vi "Individual Tube ON - OFF.vi"(6 "Single Tube ON/OFF":bool, 7 "Tube #":i32 min=0 max=63) -> ()   [LabVIEW 2020]
uses:
  <vilib>/DAQmx/write.llb/DAQmx Write (Digital U8 1Chan 1Samp).vi
  <vilib>/DAQmx/create/channels.llb/DAQmx Create Channel (DO-Digital Output).vi
  <vilib>/DAQmx/miscellaneous.llb/DAQmx Fill In Error Info.vi
panel:
  out "Status(U8) 2":u8
  in  "lines 2":tag="Dev2/port0/line0:7"
  out "Status(U8)":u8
  in  "lines":tag="Dev2/port0/line0:7"
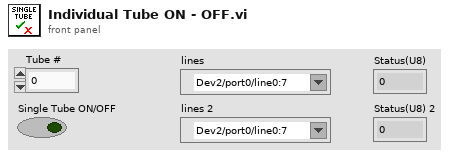
[diagram p1: front panel]
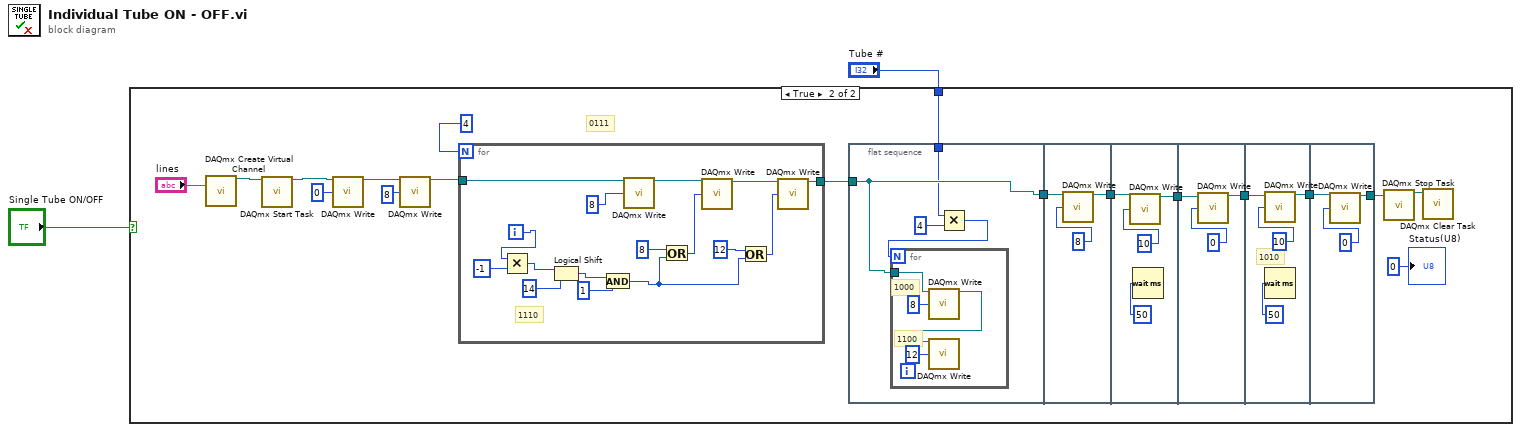
[diagram p0: block diagram]
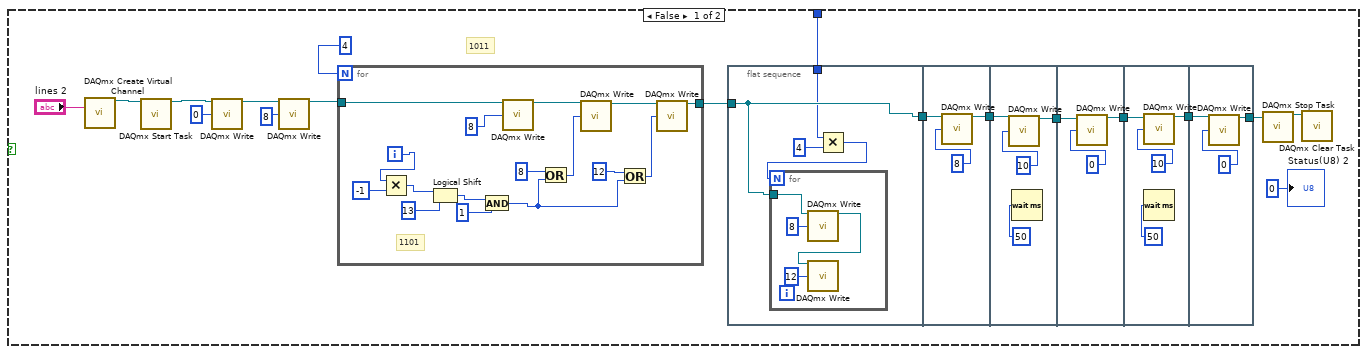
[diagram p2: hidden frame]
diagram:
  n1 = case shown="True" "Single Tube ON/OFF" {
    tunnel: "Tube #" -> [w3 w62]
    frame False {
      # "1011"
      n2 = call-poly <vilib>:"DAQmx Create Virtual Channel.vi"("lines"="lines 2") -> ("task out"=w15:refnum<k21>)  [unwired: 13 in, 1 out]
      n3 = call <vilib>:"DAQmx Start Task.vi"("task/channels in"=w15) -> ("task out"=w9:refnum<k21>)  [unwired: 13 in, 1 out]
      n4 = call-poly <vilib>:"DAQmx Write.vi"("task/channels in"=w9, "data"=u8 0) -> ("task out"=w8:refnum<k21>)  [unwired: 11 in, 2 out]
      n5 = call-poly <vilib>:"DAQmx Write.vi"("task/channels in"=w8, "data"=u8 8) -> ("task out"=w11:refnum<k21>)  [unwired: 11 in, 2 out]
      n6 = for {
        N: 4 -> [_]
        tunnel: w11 -> [w50]
        tunnel: [w47] -> w5
        i -> [w59]
        # "1101"
        n7 = Multiply(x=w59, y=-1) -> (x*y=w57:i32)
        n8 = Logical Shift(y=w57, x=u8 13) -> (x << y=w61:u8)
        n9 = And(x=w61, y=u32 1) -> (x .and. y?=w53:u32)
        n10 = call-poly <vilib>:"DAQmx Write.vi"("task/channels in"=w50, "data"=u32 8 ("x")) -> ("task out"=w49:refnum<k21>)  [unwired: 11 in, 2 out]
        n11 = Or(x=u32 8, y=w53) -> (x .or. y?=w54:u32)
        n12 = call-poly <vilib>:"DAQmx Write.vi"("task/channels in"=w49, "data"=w54) -> ("task out"=w48:refnum<k21>)  [unwired: 11 in, 2 out]
        n13 = Or(x=u32 12, y=w53) -> (x .or. y?=w51:u32)
        n14 = call-poly <vilib>:"DAQmx Write.vi"("task/channels in"=w48, "data"=w51) -> ("task out"=w47:refnum<k21>)  [unwired: 11 in, 2 out]
      }
      n15 = flat-sequence {
        tunnel: [w22] -> w20
        tunnel: w5 -> [w22]
        tunnel: w3 -> [w21]
        tunnel: [w29] -> w19
        tunnel: w20 -> [w30]
        tunnel: w19 -> [w33]
        tunnel: [w32] -> w18
        tunnel: w18 -> [w37]
        tunnel: [w36] -> w17
        tunnel: w17 -> [w40]
        tunnel: [w39] -> w16
        tunnel: w16 -> [w44]
        tunnel: [w43] -> w6
        frame #0 {
          n16 = Multiply(x=w21, y=4) -> (x*y=w24:i32)
          n17 = for {
            N: w24 -> [_]
            tunnel: w22 -> [w26]
            n18 = call-poly <vilib>:"DAQmx Write.vi"("task/channels in"=w26, "data"=u8 8) -> ("task out"=w25:refnum<k21>)  [unwired: 11 in, 2 out]
            n19 = call-poly <vilib>:"DAQmx Write.vi"("task/channels in"=w25, "data"=u8 12) -> ()  [unwired: 11 in, 3 out]
          }
        }
        frame #1 {
          n20 = call-poly <vilib>:"DAQmx Write.vi"("task/channels in"=w30, "data"=u8 8) -> ("task out"=w29:refnum<k21>)  [unwired: 11 in, 2 out]
        }
        frame #2 {
          n21 = call-poly <vilib>:"DAQmx Write.vi"("task/channels in"=w33, "data"=u8 10) -> ("task out"=w32:refnum<k21>)  [unwired: 11 in, 2 out]
          n22 = Wait (ms)(milliseconds to wait=u32 50) -> ()  [unwired: 1 out]
        }
        frame #3 {
          n23 = call-poly <vilib>:"DAQmx Write.vi"("task/channels in"=w37, "data"=u8 0) -> ("task out"=w36:refnum<k21>)  [unwired: 11 in, 2 out]
        }
        frame #4 {
          n24 = call-poly <vilib>:"DAQmx Write.vi"("task/channels in"=w40, "data"=u8 10) -> ("task out"=w39:refnum<k21>)  [unwired: 11 in, 2 out]
          n25 = Wait (ms)(milliseconds to wait=u32 50) -> ()  [unwired: 1 out]
        }
        frame #5 {
          n26 = call-poly <vilib>:"DAQmx Write.vi"("task/channels in"=w44, "data"=u8 0) -> ("task out"=w43:refnum<k21>)  [unwired: 11 in, 2 out]
        }
      }
      n27 = call <vilib>:"DAQmx Stop Task.vi"("task/channels in"=w6) -> ("task out"=w14:refnum<k21>)  [unwired: 13 in, 1 out]
      n28 = call <vilib>:"DAQmx Clear Task.vi"("task in"=w14) -> ()  [unwired: 14 in, 1 out]
      "Status(U8) 2" <- u8 0
    }
    frame True {
      # "0111"
      n29 = call-poly <vilib>:"DAQmx Create Virtual Channel.vi"("lines"="lines") -> ("task out"=w74:refnum<k21>)  [unwired: 13 in, 1 out]
      n30 = call <vilib>:"DAQmx Start Task.vi"("task/channels in"=w74) -> ("task out"=w68:refnum<k21>)  [unwired: 13 in, 1 out]
      n31 = call-poly <vilib>:"DAQmx Write.vi"("task/channels in"=w68, "data"=u8 0) -> ("task out"=w67:refnum<k21>)  [unwired: 11 in, 2 out]
      n32 = call-poly <vilib>:"DAQmx Write.vi"("task/channels in"=w67, "data"=u8 8) -> ("task out"=w70:refnum<k21>)  [unwired: 11 in, 2 out]
      n33 = for {
        N: 4 -> [_]
        tunnel: w70 -> [w109]
        tunnel: [w106] -> w64
        i -> [w118]
        # "1110"
        n34 = Multiply(x=w118, y=-1) -> (x*y=w116:i32)
        n35 = Logical Shift(y=w116, x=u8 14) -> (x << y=w120:u8)
        n36 = And(x=w120, y=u32 1) -> (x .and. y?=w112:u32)
        n37 = call-poly <vilib>:"DAQmx Write.vi"("task/channels in"=w109, "data"=u32 8 ("x")) -> ("task out"=w108:refnum<k21>)  [unwired: 11 in, 2 out]
        n38 = Or(x=u32 8, y=w112) -> (x .or. y?=w113:u32)
        n39 = call-poly <vilib>:"DAQmx Write.vi"("task/channels in"=w108, "data"=w113) -> ("task out"=w107:refnum<k21>)  [unwired: 11 in, 2 out]
        n40 = Or(x=u32 12, y=w112) -> (x .or. y?=w110:u32)
        n41 = call-poly <vilib>:"DAQmx Write.vi"("task/channels in"=w107, "data"=w110) -> ("task out"=w106:refnum<k21>)  [unwired: 11 in, 2 out]
      }
      n42 = flat-sequence {
        tunnel: [w81] -> w79
        tunnel: w64 -> [w81]
        tunnel: w62 -> [w80]
        tunnel: [w88] -> w78
        tunnel: w79 -> [w89]
        tunnel: w78 -> [w92]
        tunnel: [w91] -> w77
        tunnel: w77 -> [w96]
        tunnel: [w95] -> w76
        tunnel: w76 -> [w99]
        tunnel: [w98] -> w75
        tunnel: w75 -> [w103]
        tunnel: [w102] -> w65
        frame #0 {
          n43 = Multiply(x=w80, y=4) -> (x*y=w83:i32)
          n44 = for {
            N: w83 -> [_]
            tunnel: w81 -> [w85]
            # "1100"
            # "1000"
            n45 = call-poly <vilib>:"DAQmx Write.vi"("task/channels in"=w85, "data"=u8 8) -> ("task out"=w84:refnum<k21>)  [unwired: 11 in, 2 out]
            n46 = call-poly <vilib>:"DAQmx Write.vi"("task/channels in"=w84, "data"=u8 12) -> ()  [unwired: 11 in, 3 out]
          }
        }
        frame #1 {
          n47 = call-poly <vilib>:"DAQmx Write.vi"("task/channels in"=w89, "data"=u8 8) -> ("task out"=w88:refnum<k21>)  [unwired: 11 in, 2 out]
        }
        frame #2 {
          n48 = call-poly <vilib>:"DAQmx Write.vi"("task/channels in"=w92, "data"=u8 10) -> ("task out"=w91:refnum<k21>)  [unwired: 11 in, 2 out]
          n49 = Wait (ms)(milliseconds to wait=u32 50) -> ()  [unwired: 1 out]
        }
        frame #3 {
          n50 = call-poly <vilib>:"DAQmx Write.vi"("task/channels in"=w96, "data"=u8 0) -> ("task out"=w95:refnum<k21>)  [unwired: 11 in, 2 out]
        }
        frame #4 {
          # "1010"
          n51 = call-poly <vilib>:"DAQmx Write.vi"("task/channels in"=w99, "data"=u8 10) -> ("task out"=w98:refnum<k21>)  [unwired: 11 in, 2 out]
          n52 = Wait (ms)(milliseconds to wait=u32 50) -> ()  [unwired: 1 out]
        }
        frame #5 {
          n53 = call-poly <vilib>:"DAQmx Write.vi"("task/channels in"=w103, "data"=u8 0) -> ("task out"=w102:refnum<k21>)  [unwired: 11 in, 2 out]
        }
      }
      n54 = call <vilib>:"DAQmx Stop Task.vi"("task/channels in"=w65) -> ("task out"=w73:refnum<k21>)  [unwired: 13 in, 1 out]
      n55 = call <vilib>:"DAQmx Clear Task.vi"("task in"=w73) -> ()  [unwired: 14 in, 1 out]
      "Status(U8)" <- u8 0
    }
  }
